vi "testError.vi"() -> ()   [LabVIEW 2019, in "AssertionTest.lvlib" / "AssertNotCount.lvlib"]
uses:
  AssertNotCount.lvlib
  <vilib>/Utility/error.llb/Error Cluster From Error Code.vi
  <vilib>/ErrorRing/Error Ring.xnode
  Assertion/Assertion.lvlib
panel:
  out "error out":errorcluster
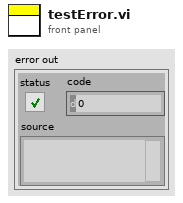
[diagram p1: front panel]
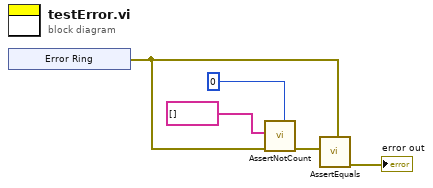
[diagram p0: block diagram]
diagram:
  n1 = xnode "Error Ring"() -> ("error out"=w1:errorcluster)
  n2 = call "AssertNotCount.vi"("Expected"=0, "error in (no error)"=w1, "Haystack"=string[] []) -> ("error out"=w3:errorcluster)  [unwired: 8 in]
  n3 = call "AssertEquals.vi"("Expected"=w1, "Actual"=w3) -> ("error out"=→"error out":errorcluster)  [unwired: 9 in]
